vi "Convert NT String to LV String.vi"(11 "Buffer in":string) -> (1 "Size":i32=1, 2 "String Contents":string, 3 "Remaining String":string)   [LabVIEW 2017]
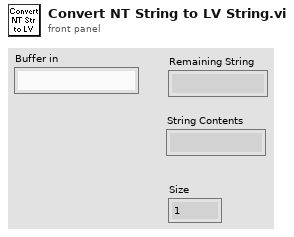
[diagram p1: front panel]
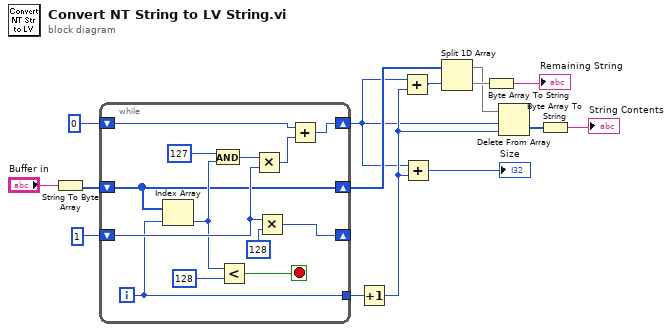
[diagram p0: block diagram]
diagram:
  n1 = String To Byte Array(string="Buffer in") -> (unsigned byte array=w10:u8[])
  n2 = while {
    shift-right: [w27] -> w1
    shift-left: u32 0 -> [w28]
    shift-right: [w25] -> _
    shift-left: u32 1 -> [w26]
    tunnel: [w17] -> w14
    shift-right: [w16] -> w6
    shift-left: w10 -> [w16]
    i -> [w17]
    stop <- w21 stop-if-true
    n3 = Index Array(array=w16, index=w17) -> (element=w18:u8)
    n4 = And(x=u8 127, y=w18) -> (x .and. y?=w20:u8)
    n5 = Less?(x=w18, y=u32 128) -> (x < y?=w21:bool)
    n6 = Multiply(x=w20, y=w26) -> (x*y=w23:u32)
    n7 = Multiply(x=w26, y=u32 128) -> (x*y=w25:u32)
    n8 = Add(x=w28, y=w23) -> (x+y=w27:u32)
  }
  n9 = Increment(x=w14) -> (x+1=w2:i32)
  n10 = Add(x=w1, y=w2) -> (x+y=w3:u32)
  n11 = Add(x=w1, y=w2) -> (x+y=→"Size":u32)
  n12 = Split 1D Array(array=w6, index=w3) -> (first subarray=w4:u8[], second subarray=w5:u8[])
  n13 = Byte Array To String(unsigned byte array=w5) -> (string=→"Remaining String":string)
  n14 = Delete From Array(array=w4, length=w1, index=w2) -> (deleted portion=w8:u8[])  [unwired: 1 out]
  n15 = Byte Array To String(unsigned byte array=w8) -> (string=→"String Contents":string)
